vi "H5Dwrite (Variant).vi"(4 "Data":variant, 5 "HDF5 File Space Ref (H5S_ALL)":T1, 6 "HDF5 Property List Ref (H5P_DEFAULT)":T1, 7 "HDF5 Memory Space Ref (H5S_ALL)":T1, 8 "error in (no error)":errorcluster, 10 "HDF5 Type Ref (match data)":T1, 11 "HDF5 Dataset Ref":T1) -> (0 "error out":errorcluster, 3 "HDF5 Ref out":T1)   [LabVIEW 2017]
doc: "Writes raw data from a buffer to a dataset."
uses:
  <vilib>/UPVI/lvhdf5/library.llb/HDF5 Ref.ctl
  <vilib>/UPVI/lvhdf5/error.llb/LVH5EMajorID.ctl
  <vilib>/UPVI/lvhdf5/error.llb/LVH5EMinorID.ctl
  <vilib>/UPVI/lvhdf5/identifier.llb/H5Iget_type.vi
  <vilib>/UPVI/lvhdf5/h5helper.dll
panel:
  # "LVHDF5 Toolkit\nCopyright (c) 2005-2013 by Jason D. Sommerville\nCopyright (c) 2014 by UPVI, LLC.\n\nThis use and distribution of this file is governed by the terms found in \nLICENSE.txt distributed with this toolkit and installed at\n <user.lib>\\_lvhdf5\\LICENSE.txt"
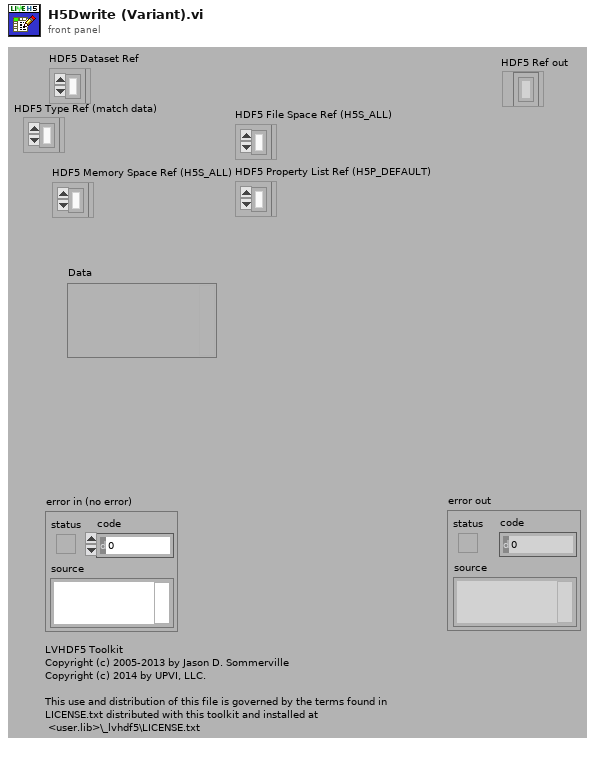
[diagram p1: front panel]
types:
  T1 = typedef "HDF5 Ref.ctl" = refnum<k1>
  T2 = typedef "LVH5EMinorID.ctl" = string
  T3 = typedef "LVH5EMajorID.ctl" = string
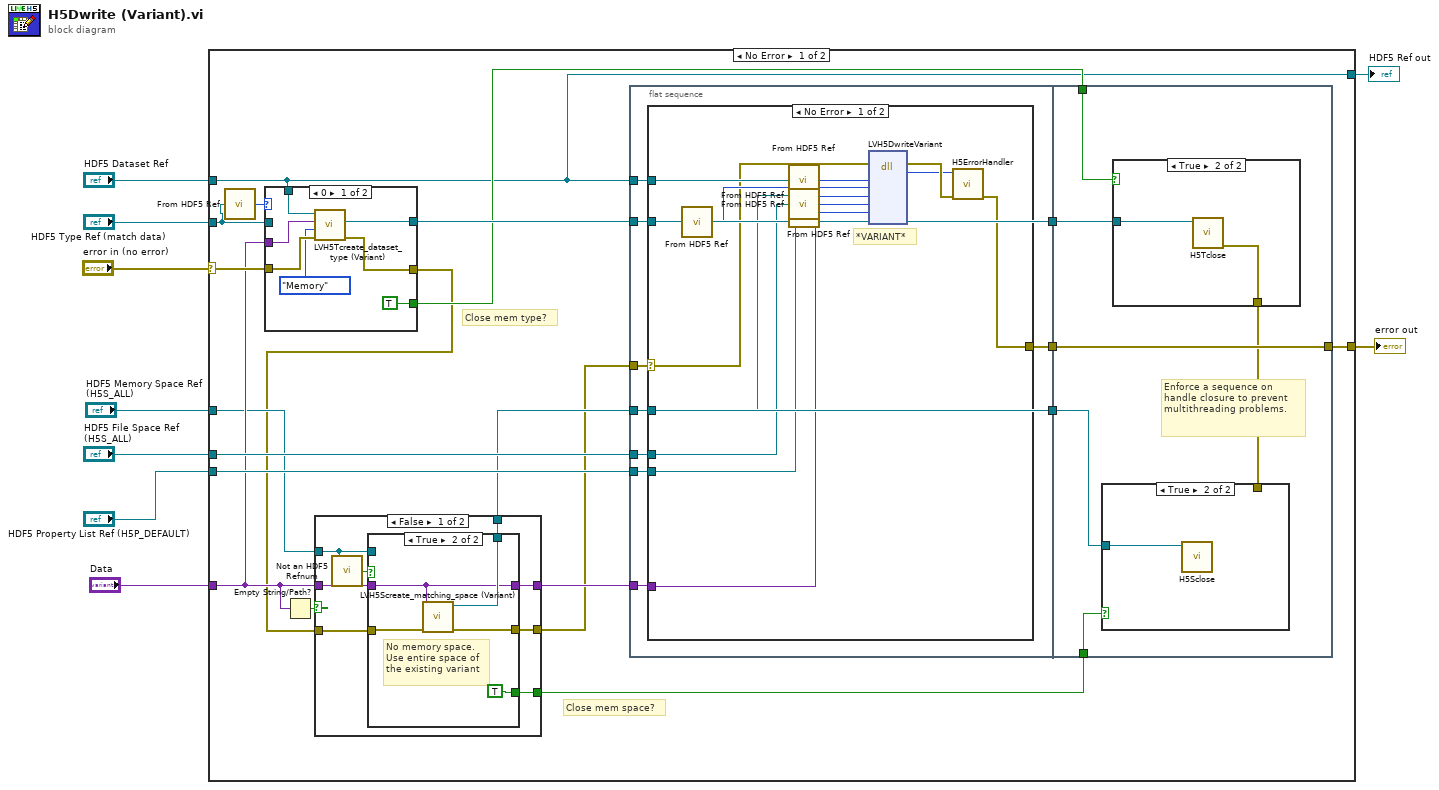
[diagram p0: block diagram]
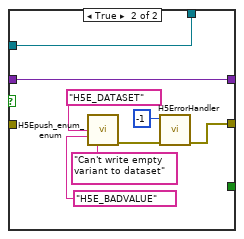
[diagram p3: hidden frame]
diagram:
  n1 = case shown="No Error" "error in (no error)" {
    selector: "error in (no error)" -> [w28 w97]
    tunnel: [w25 w97] -> w8
    tunnel: "HDF5 Dataset Ref" -> [w13 w96]
    tunnel: "HDF5 Property List Ref (H5P_DEFAULT)" -> [w26 _]
    tunnel: "HDF5 File Space Ref (H5S_ALL)" -> [w29 _]
    tunnel: "HDF5 Memory Space Ref (H5S_ALL)" -> [w20 _]
    tunnel: "Data" -> [w22 _]
    tunnel: "HDF5 Type Ref (match data)" -> [w24 _]
    tunnel: [w13 w96] -> w1
    frame No Error {
      # "Close mem space?"
      # "Close mem type?"
      n2 = call <vilib>:"From HDF5 Ref.vi"("HDF5 Ref"=w24) -> ("I32"=w23:i32)
      n3 = case shown="0" w23 {
        tunnel: [w89 w95] -> w27
        tunnel: w13 -> [w93 _]
        tunnel: w22 -> [w92 _]
        tunnel: w28 -> [w91 w94]
        tunnel: w24 -> [_ w95]
        tunnel: [w88 w94] -> w11
        tunnel: [TRUE _] -> w17
        frame 0 {
          n4 = call <vilib>:"LVH5Tcreate_dataset_type (Variant).vi"("error in (no error)"=w91, "Type"=enum16{"File", "Memory"}."Memory", "Data"=w92, "HDF5 Ref"=w93) -> ("error out"=w88:errorcluster, "HDF5 Type Ref"=w89:T1)  [unwired: 3 in, 3 out]
        }
        frame 1, Default {
        }
      }
      n5 = Empty String/Path?(string/path=w22) -> (empty?=w12:bool)
      n6 = case shown="False" w12 {
        tunnel: w22 -> [w36 w52]
        tunnel: w20 -> [w32 w53]
        tunnel: [w35 w46] -> w10
        tunnel: [w34 w53] -> w19
        tunnel: [w33 w52] -> w21
        tunnel: [w31 _] -> w14
        tunnel: w11 -> [w30 _]
        frame False {
          n7 = call <vilib>:"Not an HDF5 Refnum.vi"("HDF5 Ref"=w32) -> ("Not an HDF5 Refnum"=w37:bool)
          n8 = case shown="True" w37 {
            tunnel: w36 -> [w39 w43]
            tunnel: [w38 w45] -> w35
            tunnel: [w40 w44] -> w34
            tunnel: [w39 w43] -> w33
            tunnel: w32 -> [w40 _]
            tunnel: [_ TRUE] -> w31
            tunnel: w30 -> [w38 w41]
            frame False {
              # "Memory space\nspecified.\nSomething in _Data.\nHopefully they work together, but it's out of our hands."
            }
            frame True {
              # "No memory space.\nUse entire space of \nthe existing variant"
              n9 = call <vilib>:"LVH5Screate_matching_space (Variant).vi"("error in (no error)"=w41, "Data"=w43) -> ("error out"=w45:errorcluster, "HDF5 Dataspace Ref"=w44:T1)  [unwired: 6 in]
            }
          }
        }
        frame True {
          n10 = call <vilib>:"H5Epush_enum_enum.vi"("major_id"=T3 "H5E_DATASET", "minor_id"=T2 "H5E_BADVALUE", "msg"="Can't write empty variant to dataset") -> ("error out"=w48:errorcluster)  [unwired: 11 in, 1 out]
          n11 = call <vilib>:"H5ErrorHandler.vi"("error in (no error)"=w48, "herr_t"=-1) -> ("error out"=w46:errorcluster)  [unwired: 3 in, 4 out]
        }
      }
      n12 = flat-sequence {
        tunnel: w29 -> [w61]
        tunnel: w27 -> [w55]
        tunnel: w26 -> [w60]
        tunnel: w13 -> [w58]
        tunnel: w21 -> [w57]
        tunnel: w19 -> [w54]
        tunnel: w10 -> [w56]
        tunnel: [w59] -> w18
        tunnel: [w55] -> w16
        tunnel: [w54] -> w15
        tunnel: [w83] -> w25
        tunnel: w18 -> [w83]
        tunnel: w17 -> [w82]
        tunnel: w16 -> [w81]
        tunnel: w15 -> [w80]
        tunnel: w14 -> [w79]
        frame #0 {
          n13 = case shown="No Error" w56 {
            selector: w56 -> [w62 w77]
            tunnel: w57 -> [w66 _]
            tunnel: w54 -> [w71 _]
            tunnel: w61 -> [w70 _]
            tunnel: w58 -> [w72 _]
            tunnel: w55 -> [w68 _]
            tunnel: w60 -> [w69 _]
            tunnel: [w65 w77] -> w59
            frame No Error {
              # "*VARIANT*"
              n14 = call <vilib>:"From HDF5 Ref.vi"("HDF5 Ref"=w68) -> ("I32"=w67:i32)
              n15 = call <vilib>:"From HDF5 Ref.vi"("HDF5 Ref"=w72) -> ("I32"=w75:i32)
              n16 = call <vilib>:"From HDF5 Ref.vi"("HDF5 Ref"=w71) -> ("I32"=w63:i32)
              n17 = call <vilib>:"From HDF5 Ref.vi"("HDF5 Ref"=w70) -> ("I32"=w74:i32)
              n18 = call <vilib>:"From HDF5 Ref.vi"("HDF5 Ref"=w69) -> ("I32"=w73:i32)
              n19 = dll-call lib="C:/Program Files/National Instruments/LabVIEW 2017/vi.lib/UPVI/lvhdf5/h5helper.dll" fn="LVH5DwriteVariant"(error in=w62, "dataset_id"=w75, "mem_type_id"=w67, "mem_space_id"=w63, "file_space_id"=w74, "xfer_plist_id"=w73, "buf"=w66) -> (error out=w76:errorcluster, "return type"=w64:i32)  [unwired: 8 in, 1 out]
              n20 = call <vilib>:"H5ErrorHandler.vi"("error in (no error)"=w76, "herr_t"=w64) -> ("error out"=w65:errorcluster)  [unwired: 3 in, 4 out]
            }
            frame Error {
            }
          }
        }
        frame #1 {
          # "Enforce a sequence on handle closure to prevent multithreading problems."
          n21 = case shown="True" w82 {
            tunnel: w81 -> [_ w86]
            tunnel: [_ w85] -> w78
            frame False {
            }
            frame True {
              n22 = call <vilib>:"H5Tclose.vi"("HDF5 Datatype Ref"=w86) -> ("error out"=w85:errorcluster)  [unwired: 8 in]
            }
          }
          n23 = case shown="True" w79 {
            tunnel: w80 -> [_ w84]
            tunnel: w78 -> [_ _]
            frame False {
            }
            frame True {
              n24 = call <vilib>:"H5Sclose.vi"("HDF5 Dataspace Ref"=w84) -> ()  [unwired: 8 in, 1 out]
            }
          }
        }
      }
    }
    frame Error {
    }
  }
  "error out" <- w8
  "HDF5 Ref out" <- w1
